vi "serial read.vi"(8 "error in (no error)":errorcluster, 10 "opMode":enum16{"default", "injector", "gas analyzer"}(ring), 11 "VISA resource name in":refnum<visa-resource-name>) -> (0 "error out":errorcluster, 1 "bytes count":u32, 2 "read buffer":string, 3 "VISA resource name out":refnum<visa-resource-name>)   [LabVIEW 2016]
uses:
  <vilib>/Instr/_visa.llb/VISA Flush IO Buffer Mask.ctl
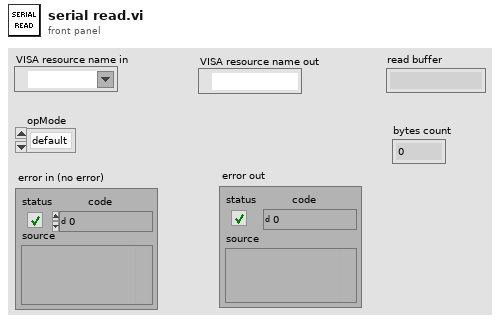
[diagram p1: front panel]
types:
  T1 = typedef "VISA Flush IO Buffer Mask.ctl" = u16
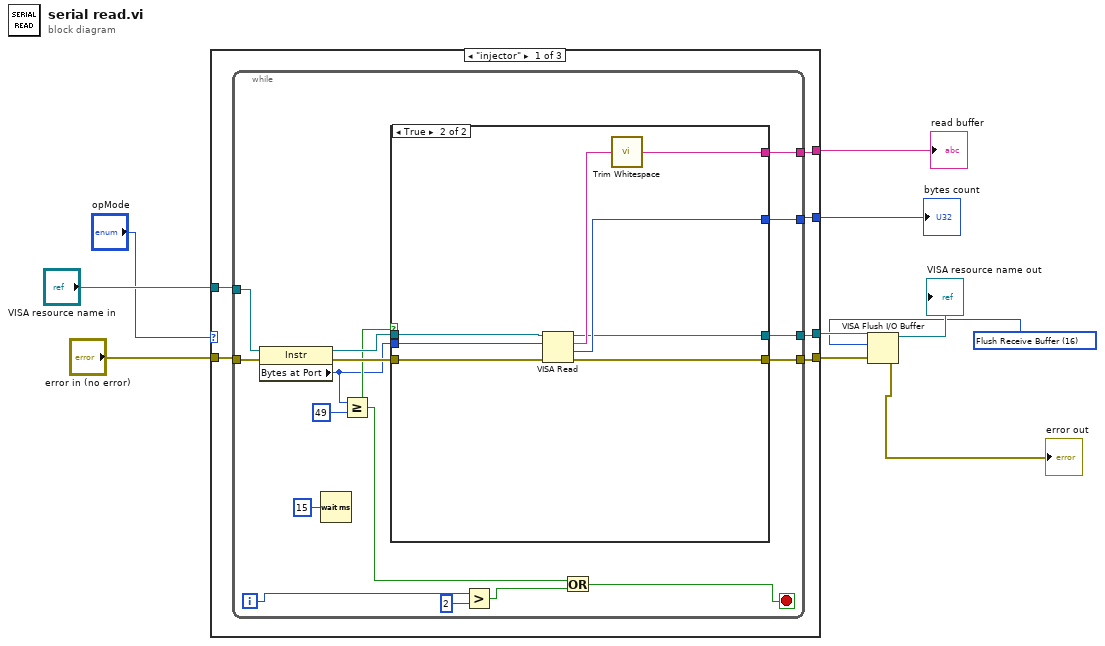
[diagram p0: block diagram]
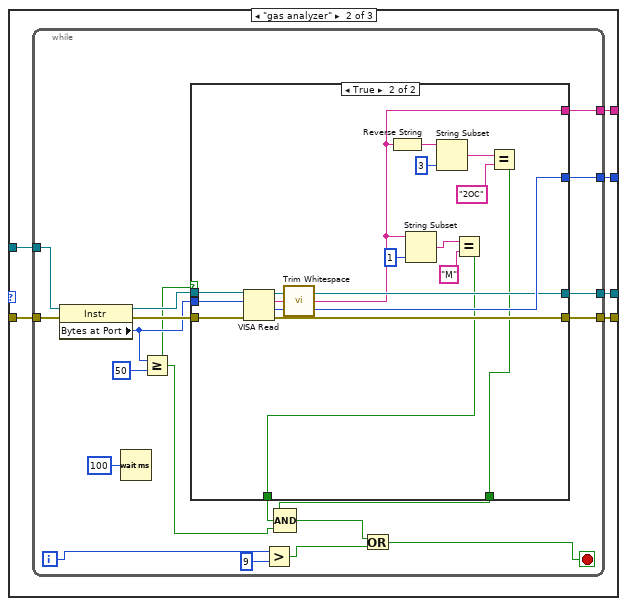
[diagram p3: hidden frame]
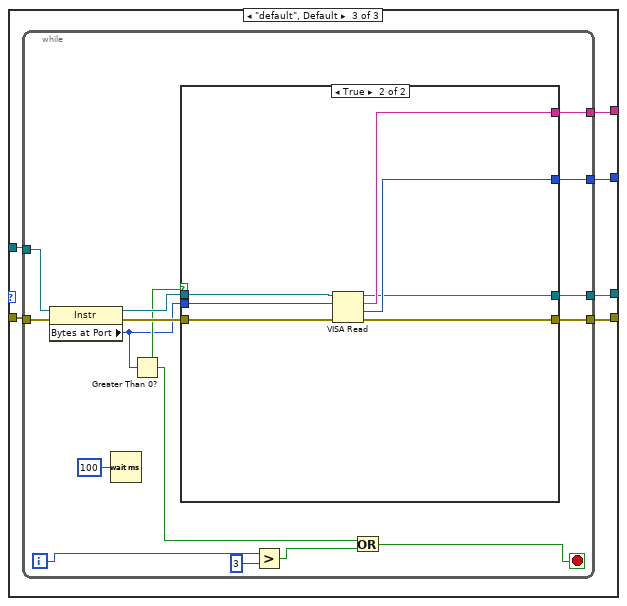
[diagram p5: hidden frame]
diagram:
  w3 = T1 16 items=["Flush Receive Buffer"=16, "Write Transmit Buffer to Device"=32, "Flush Receive Buffer (No I/O)"=64, "Flush Transmit Buffer"=128] ("Mask")
  n1 = case shown="\"injector\"" "opMode" {
    tunnel: "VISA resource name in" -> [w16 w49 w94]
    tunnel: "error in (no error)" -> [w15 w48 w93]
    tunnel: [w14 w47 w92] -> w8
    tunnel: [w13 w46 w91] -> w7
    tunnel: [w12 w45 w90] -> w6
    tunnel: [w11 w44 w89] -> w5
    frame "injector" {
      n2 = while {
        tunnel: w16 -> [w32]
        tunnel: w15 -> [w31]
        tunnel: [w30] -> w14
        tunnel: [w29] -> w13
        tunnel: [w28] -> w12
        tunnel: [w27] -> w11
        i -> [w21]
        stop <- w19 stop-if-true
        n3 = property class="Instr"(reference=w32, error in=w31) -> (reference out=w25:refnum<visa-resource-name>, error out=w26:errorcluster, "Bytes at Port"=w18:u32)
        n4 = Wait (ms)(milliseconds to wait=u32 15) -> ()  [unwired: 1 out]
        n5 = Greater Or Equal?(x=w18, y=u32 49) -> (x >= y?=w23:bool)
        n6 = case shown="True" w23 {
          tunnel: [_ w36] -> w30
          tunnel: [w33 w42] -> w29
          tunnel: [w35 w41] -> w28
          tunnel: [w34 w40] -> w27
          tunnel: w26 -> [w34 w39]
          tunnel: w18 -> [w33 w38]
          tunnel: w25 -> [w35 w37]
          frame False {
          }
          frame True {
            n7 = VISA Read(VISA resource name=w37, byte count=w38, error in (no error)=w39) -> (VISA resource name out=w41:refnum<visa-resource-name>, read buffer=w43:string, return count=w42:u32, error out=w40:errorcluster)
            n8 = call <vilib>:"Trim Whitespace.vi"("string"=w43) -> ("trimmed string"=w36:string)  [unwired: 1 in]
          }
        }
        n9 = Greater?(x=w21, y=2) -> (0:w22:bool)
        n10 = Or(x=w23, y=w22) -> (x .or. y?=w19:bool)
      }
    }
    frame "gas analyzer" {
      n11 = while {
        tunnel: w49 -> [w68]
        tunnel: w48 -> [w67]
        tunnel: [w66] -> w47
        tunnel: [w65] -> w46
        tunnel: [w64] -> w45
        tunnel: [w63] -> w44
        i -> [w58]
        stop <- w56 stop-if-true
        n12 = property class="Instr"(reference=w68, error in=w67) -> (reference out=w61:refnum<visa-resource-name>, error out=w62:errorcluster, "Bytes at Port"=w55:u32)
        n13 = Wait (ms)(milliseconds to wait=u32 100) -> ()  [unwired: 1 out]
        n14 = Greater Or Equal?(x=w55, y=u32 50) -> (x >= y?=w53:bool)
        n15 = case shown="True" w53 {
          tunnel: [_ w72] -> w66
          tunnel: [w69 w88] -> w65
          tunnel: [w71 w87] -> w64
          tunnel: [w70 w86] -> w63
          tunnel: w62 -> [w70 w85]
          tunnel: w55 -> [w69 w84]
          tunnel: w61 -> [w71 w83]
          tunnel: [_ w74] -> w52
          tunnel: [_ w73] -> w51
          frame False {
          }
          frame True {
            n16 = VISA Read(VISA resource name=w83, byte count=w84, error in (no error)=w85) -> (VISA resource name out=w87:refnum<visa-resource-name>, read buffer=w79:string, return count=w88:u32, error out=w86:errorcluster)
            n17 = call <vilib>:"Trim Whitespace.vi"("string"=w79) -> ("trimmed string"=w72:string)  [unwired: 1 in]
            n18 = Reverse String(1:w72) -> (0:w78:string)
            n19 = String Subset(string=w72, length (rest)=1 ("length (rest)")) -> (substring=w81:string)  [unwired: 1 in]
            n20 = String Subset(string=w78, length (rest)=3 ("length (rest)")) -> (substring=w76:string)  [unwired: 1 in]
            n21 = Equal?(x=w81, y="M") -> (x = y?=w74:bool)
            n22 = Equal?(x=w76, y="2OC") -> (x = y?=w73:bool)
          }
        }
        n23 = Greater?(x=w58, y=9) -> (0:w59:bool)
        n24 = Compound Arithmetic op=AND(w51, w52, w53) -> (w50:bool)
        n25 = Or(x=w50, y=w59) -> (x .or. y?=w56:bool)
      }
    }
    frame "default", Default {
      n26 = while {
        tunnel: w94 -> [w109]
        tunnel: w93 -> [w108]
        tunnel: [w107] -> w92
        tunnel: [w106] -> w91
        tunnel: [w105] -> w90
        tunnel: [w104] -> w89
        i -> [w98]
        stop <- w96 stop-if-true
        n27 = property class="Instr"(reference=w109, error in=w108) -> (reference out=w102:refnum<visa-resource-name>, error out=w103:errorcluster, "Bytes at Port"=w95:u32)
        n28 = Wait (ms)(milliseconds to wait=u32 100) -> ()  [unwired: 1 out]
        n29 = Greater Than 0?(x=w95) -> (x > 0?=w100:bool)
        n30 = case shown="True" w100 {
          tunnel: [_ w119] -> w107
          tunnel: [w110 w118] -> w106
          tunnel: [w112 w117] -> w105
          tunnel: [w111 w116] -> w104
          tunnel: w103 -> [w111 w115]
          tunnel: w95 -> [w110 w114]
          tunnel: w102 -> [w112 w113]
          frame False {
          }
          frame True {
            n31 = VISA Read(VISA resource name=w113, byte count=w114, error in (no error)=w115) -> (VISA resource name out=w117:refnum<visa-resource-name>, read buffer=w119:string, return count=w118:u32, error out=w116:errorcluster)
          }
        }
        n32 = Greater?(x=w98, y=3) -> (0:w99:bool)
        n33 = Or(x=w100, y=w99) -> (x .or. y?=w96:bool)
      }
    }
  }
  "read buffer" <- w8
  "bytes count" <- w7
  n34 = VISA Flush I/O Buffer(VISA resource name=w6, mask (16)=w3, error in (no error)=w5) -> (VISA resource name out=→"VISA resource name out":refnum<visa-resource-name>, error out=→"error out":errorcluster)
